vi "Build report string.vi"(8 "error in (no error)":errorcluster, 11 "Work period":T1[](array[typedef])) -> (0 "error out":errorcluster, 3 "Report string":string)   [LabVIEW 2015]
uses:
  DatabaseManager/WorkDay.ctl
panel:
  # "Connector Pane"
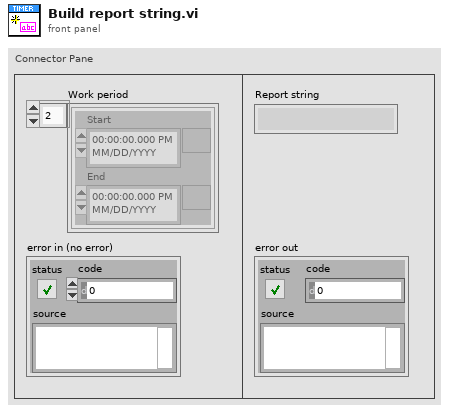
[diagram p1: front panel]
types:
  T1 = typedef "WorkDay.ctl" = cluster{"Start":timestamp, "End":timestamp}
  T2 = typedef "LVDateTimeRec.ctl" = cluster{"fractional second":dbl, "second":i32, "minute":i32, "hour":i32, "day of month":i32, "month":i32, "year":i32, "day of week":i32, "day of year":i32, "DST":i32}
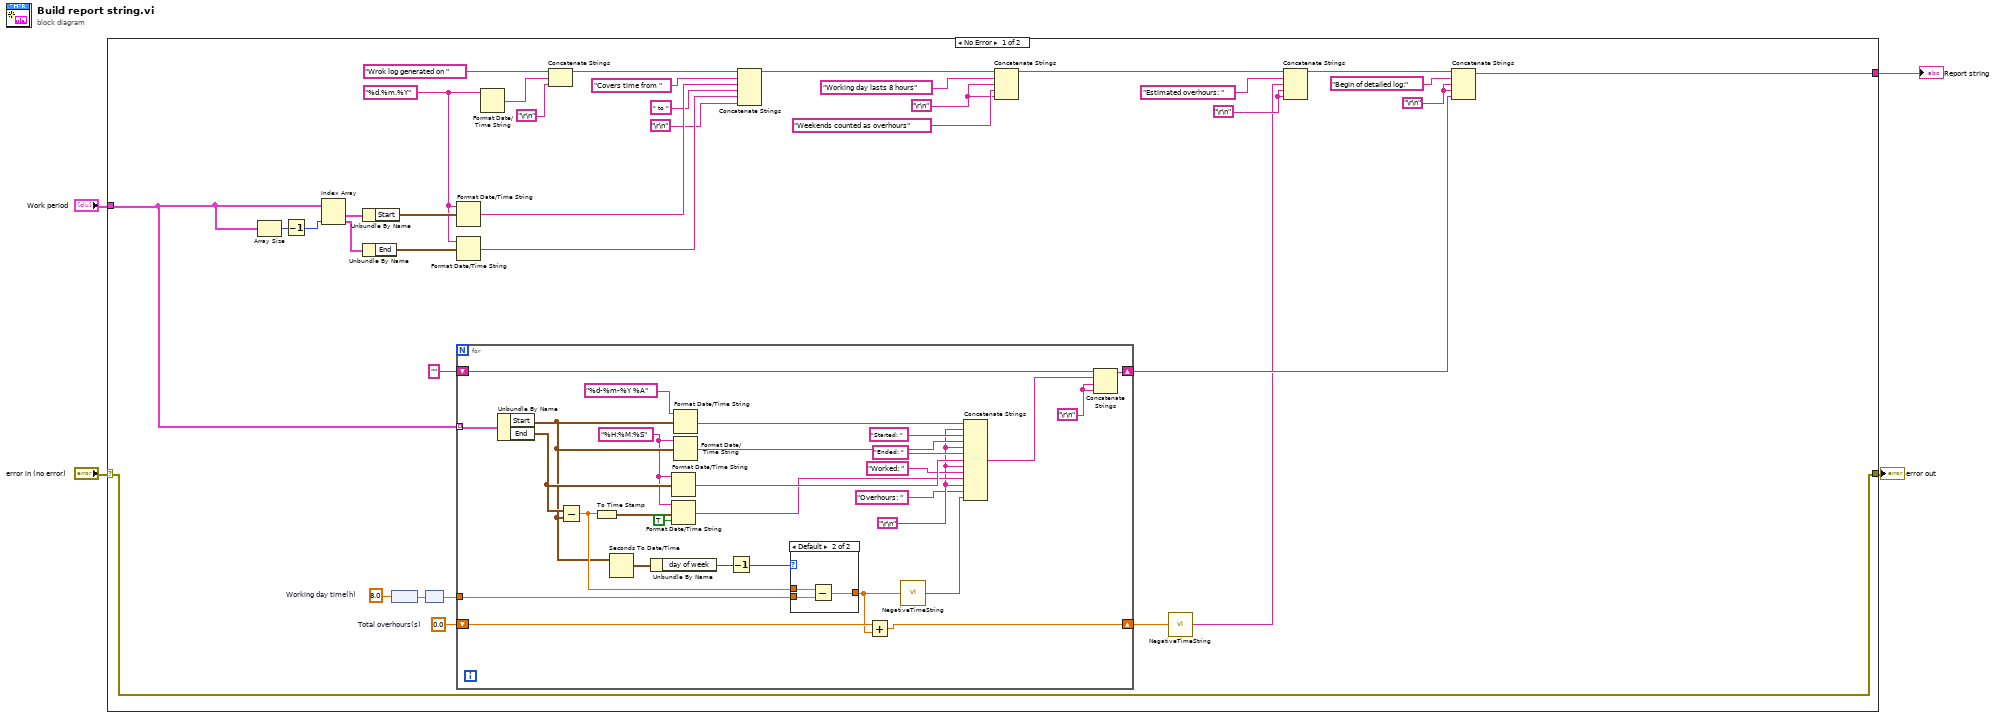
[diagram p0: block diagram]
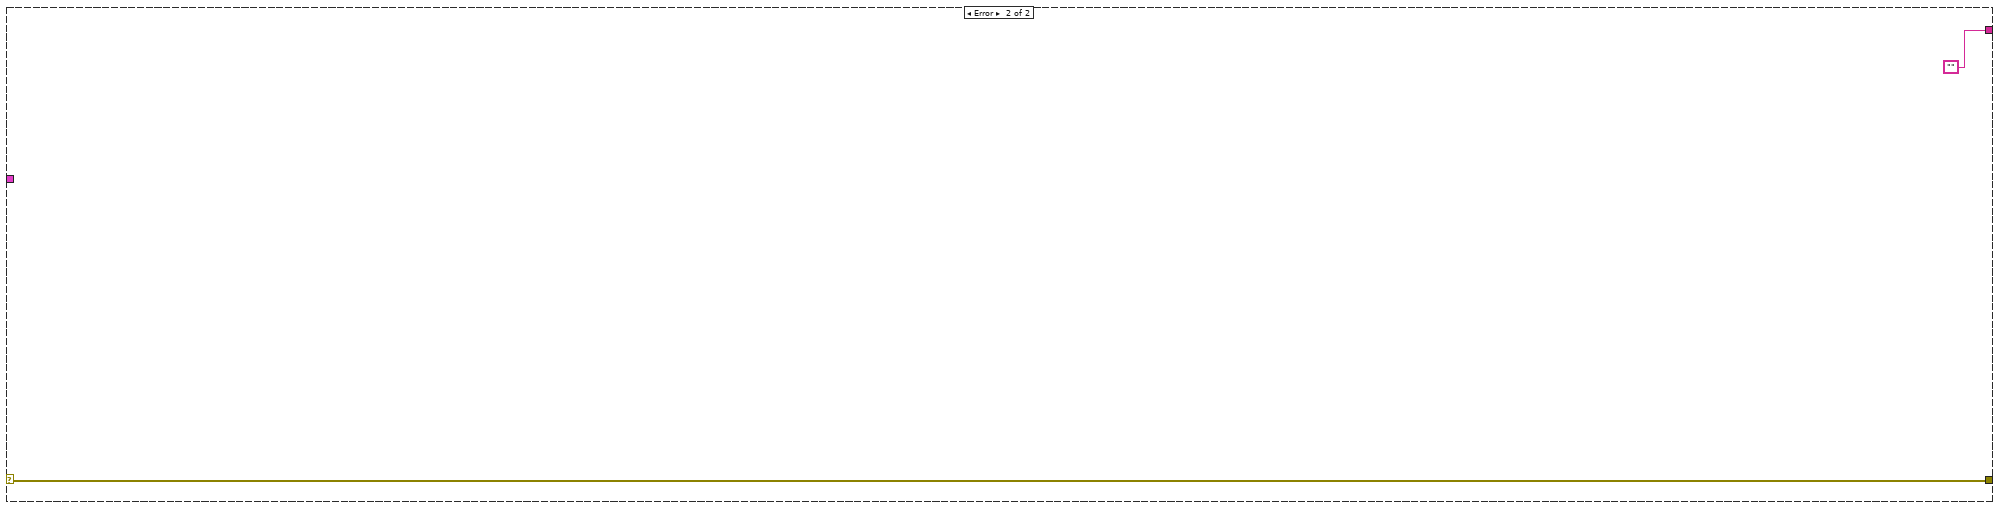
[diagram p3: hidden frame]
diagram:
  n1 = case shown="No Error" "error in (no error)" {
    selector: "error in (no error)" -> [w12 w76]
    tunnel: [w12 w76] -> w3
    tunnel: "Work period" -> [w15 _]
    tunnel: [w5 ""] -> w1
    frame No Error {
      w10 = 8.0  # Working day time(h)
      w11 = 0.0  # Total overhours(s)
      w16 = "\r\n"
      w18 = "\r\n"
      w22 = "\r\n"
      w29 = "%d.%m.%Y" ("time format string (%c)")
      n2 = Array Size(array=w15) -> (size(s)=w41:i32)
      n3 = Decrement(x=w41) -> (x-1=w40:i32)
      n4 = Index Array(array=w15, index #2=w40) -> (element #1=w39:T1, element #2=w38:T1)  [unwired: 1 in]
      n5 = Unbundle By Name(w39) -> ("Start"=w32:timestamp)
      n6 = Unbundle By Name(w38) -> ("End"=w28:timestamp)
      n7 = node(w10) -> (w9:dbl[unit])
      n8 = node(w9) -> (w8:dbl)
      n9 = Format Date/Time String(time format string (%c)=w29, seconds (now)=w32) -> (date/time string=w31:string)  [unwired: 1 in]
      n10 = Format Date/Time String(time format string (%c)=w29, seconds (now)=w28) -> (date/time string=w27:string)  [unwired: 1 in]
      n11 = for {
        tunnel: w15 -> [w70] mode=indexing
        shift-right: [w58] -> w13
        shift-left: "" -> [w59]
        shift-right: [w52] -> w7
        shift-left: w11 -> [w53]
        tunnel: w8 -> [w54]
        w42 = "\r\n"
        w45 = "%H:%M:%S" ("time format string (%c)")
        w48 = "\r\n"
        n12 = Unbundle By Name(w70) -> ("Start"=w51:timestamp, "End"=w63:timestamp)
        n13 = Subtract(x=w63, y=w51) -> (x-y=w55:dbl)
        n14 = To Time Stamp(1:w55) -> (0:w61:timestamp)
        n15 = Seconds To Date/Time(time stamp (now)=w51) -> (date time rec=w50:T2)  [unwired: 1 in]
        n16 = Unbundle By Name(w50) -> ("day of week"=w49:i32)
        n17 = Format Date/Time String(time format string (%c)=w45, seconds (now)=w63) -> (date/time string=w64:string)  [unwired: 1 in]
        n18 = Format Date/Time String(time format string (%c)=w45, seconds (now)=w61, UTC format=TRUE) -> (date/time string=w60:string)
        n19 = Format Date/Time String(time format string (%c)="%d-%m-%Y %A", seconds (now)=w51) -> (date/time string=w68:string)  [unwired: 1 in]
        n20 = Format Date/Time String(time format string (%c)=w45, seconds (now)=w51) -> (date/time string=w66:string)  [unwired: 1 in]
        n21 = Decrement(x=w49) -> (x-1=w43:i32)
        n22 = case shown="Default" w43 {
          tunnel: w55 -> [w71 w74]
          tunnel: w54 -> [_ w73]
          tunnel: [w71 w72] -> w46
          frame 6, 7 {
          }
          frame Default {
            n23 = Subtract(x=w74, y=w73) -> (x-y=w72:dbl)
          }
        }
        n24 = Add(x=w53, y=w46) -> (x+y=w52:dbl)
        n25 = call "NegativeTimeString.vi"("Time(s)"=w46) -> ("Relative time string"=w44:string)
        n26 = Concatenate Strings(w68, w48, "Started: " ("string"), w66, w48, "Ended: " ("string"), w64, w48, "Worked: " ("string"), w60, w48, "Overhours: " ("string"), w44) -> (w57:string)
        n27 = Concatenate Strings(w59, w57, w42, w42) -> (w58:string)
      }
      n28 = Format Date/Time String(time format string (%c)=w29) -> (date/time string=w36:string)  [unwired: 2 in]
      n29 = Concatenate Strings("Wrok log generated on " ("string"), w36, "\r\n") -> (w34:string)
      n30 = Concatenate Strings(w34, "Covers time from " ("string"), w31, " to " ("string"), w27, "\r\n") -> (w25:string)
      n31 = Concatenate Strings(w25, "Working day lasts 8 hours" ("string"), w22, "Weekends counted as overhours" ("string"), w22) -> (w21:string)
      n32 = call "NegativeTimeString.vi"("Time(s)"=w7) -> ("Relative time string"=w6:string)
      n33 = Concatenate Strings(w21, "Estimated overhours: " ("string"), w6, w18, w18) -> (w19:string)
      n34 = Concatenate Strings(w19, "Begin of detailed log:" ("string"), w16, w16, w13) -> (w5:string)
    }
    frame Error {
    }
  }
  "error out" <- w3
  "Report string" <- w1
